vi "water level detection system using arduino.vi"() -> ()   [LabVIEW 2022 SP3]
uses:
  <vilib>/MakerHub/LINX/Public/Peripherals/Analog/Analog Read 1 Chan.vi
  <vilib>/MakerHub/LINX/Public/Peripherals/Digital/Digital Write 1 Chan.vi
  <vilib>/MakerHub/LINX/Public/Peripherals/Analog/Analog Read N Chans.vi
  <vilib>/MakerHub/LINX/Public/Peripherals/Digital/Digital Write N Chans.vi
  <vilib>/MakerHub/LINX/Private/Local IO/LinxAnalogRead.vi
  <vilib>/MakerHub/LINX/Public/Utilities/Check Channel.vi
  <vilib>/MakerHub/LINX/Private/Local IO/LinxDigitalWrite.vi
  <vilib>/MakerHub/LINX/Public/Utilities/Open Serial.vi
  <vilib>/MakerHub/LINX/Private/Utilties/Generate Error.vi
  <vilib>/MakerHub/LINX/LMH-LINX.lvlib
panel:
  out "Boolean 4":bool
  out "Boolean 3":bool
  out "Boolean 2":bool
  out "Boolean":bool
  in  "DO Channel 4":u8
  in  "DO Channel 3":u8
  in  "DO Channel 2":u8
  in  "DO Channel":u8
  in  "stop":bool
  out "Tank":dbl(slide) scale=0.0..10.0
  out "Voltage":dbl
  in  "Analog Channel":u8
  in  "Serial Port":refnum<visa-resource-name>="N/A"
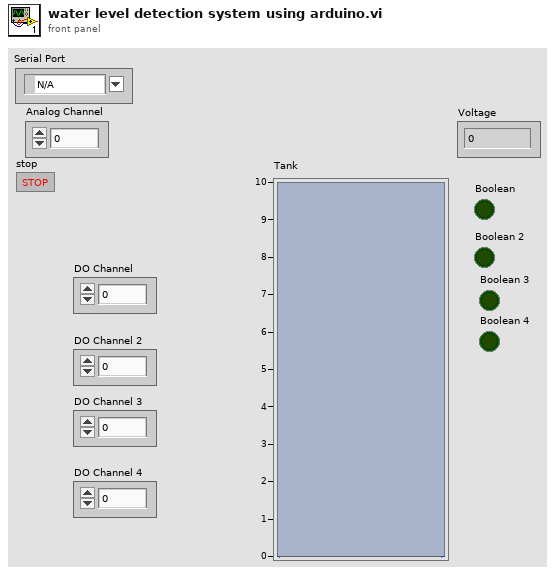
[diagram p1: front panel]
types:
  T1 = typedef "LMH-LINX.lvlib/LINX Ref.ctl" = cluster{"IO":T2, "Interface":T3, "LINX Device Config":T4}
  T2 = typedef "LMH-LINX.lvlib/Platform.ctl" = enum16{"Remote", "Local"}
  T3 = typedef "LMH-LINX.lvlib/Interface.ctl" = enum16{"Serial", "TCP"}
  T4 = typedef "LMH-LINX.lvlib/Device.lvlib/LINX Device Config.ctl" = cluster{"Interface":T3, "COM Port":refnum<visa-resource-name>, "TCP Configuration":T5, "Device Family":u8, "Device ID":u8, "Device Name":string, "TCP Ref":refnum<k5>, "Channels":T6}
  T5 = typedef "LMH-LINX.lvlib/Device.lvlib/TCP Config.ctl" = cluster{"IP Address":string, "Port":u16}
  T6 = typedef "LMH-LINX.lvlib/Channels.ctl" = cluster{"DI":u8[], "DO":u8[], "AI":u8[], "AO":u8[], "PWM":u8[], "QE":u8[], "UART":u8[], "I2C 2":u8[], "SPI":u8[], "CAN":u8[], "Servo":u8[], "AI Ref (V)":dbl, "AI Resolution (Bits)":u8, "AO Ref (V)":dbl, "AO Resolution (Bits)":u8}
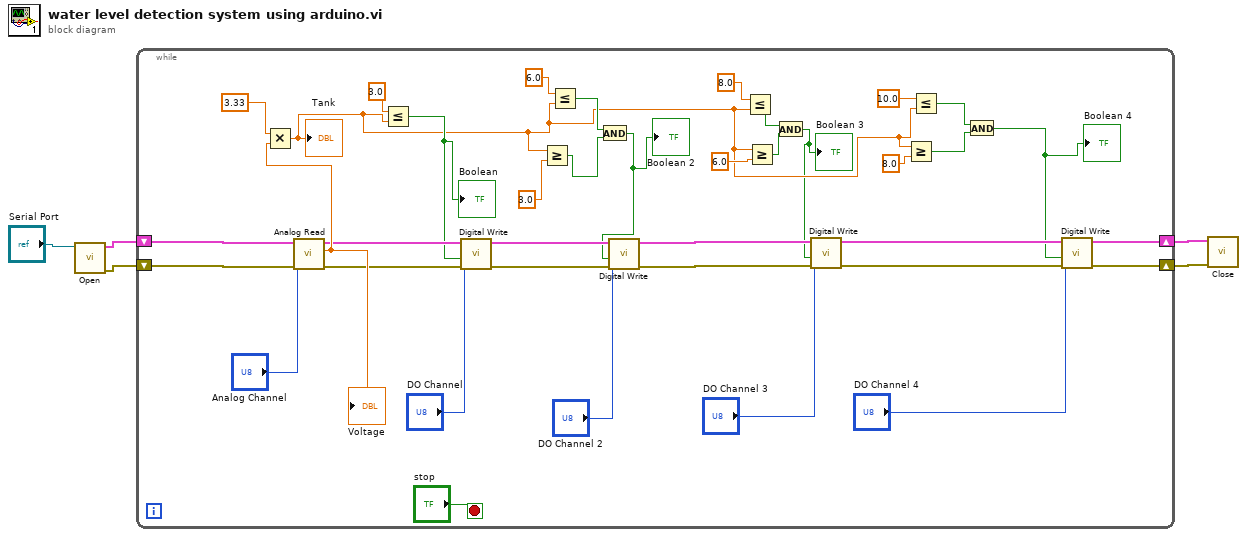
[diagram p0: block diagram]
diagram:
  n1 = call-poly <vilib>:"Open.vi"("Serial Port"="Serial Port") -> ("Error Out"=w3:errorcluster, "LINX Resource"=w4:T1)  [unwired: 8 in, 1 out]
  n2 = while {
    shift-right: [w29] -> w2
    shift-left: w4 -> [w43]
    shift-right: [w28] -> w1
    shift-left: w3 -> [w42]
    stop <- "stop" stop-if-true
    n3 = call-poly <vilib>:"Analog Read.vi"("Error In"=w42, "Analog Channel"="Analog Channel", "LINX Resource"=w43) -> ("Error Out"=w36:errorcluster, "Voltage"=w39:dbl, "LINX Resource"=w37:T1)  [unwired: 5 in, 1 out]
    "Voltage" <- w39
    n4 = Multiply(x=3.33, y=w39) -> (x*y=w10:dbl)
    "Tank" <- w10
    n5 = Less Or Equal?(x=3.0 ("first"), y=w10) -> (x <= y?=w22:bool)
    "Boolean" <- w22
    n6 = call-poly <vilib>:"Digital Write.vi"("Error In"=w36, "Output Value"=w22, "DO Channel"="DO Channel", "LINX Resource"=w37) -> ("Error Out"=w34:errorcluster, "LINX Resource"=w35:T1)  [unwired: 6 in]
    n7 = Greater Or Equal?(x=w10, y=3.0) -> (x >= y?=w18:bool)
    n8 = Less Or Equal?(x=6.0, y=w10) -> (x <= y?=w19:bool)
    n9 = And(x=w19, y=w18) -> (x .and. y?=w17:bool)
    "Boolean 2" <- w17
    n10 = call-poly <vilib>:"Digital Write.vi"("Error In"=w34, "Output Value"=w17, "DO Channel"="DO Channel 2", "LINX Resource"=w35) -> ("Error Out"=w32:errorcluster, "LINX Resource"=w33:T1)  [unwired: 6 in]
    n11 = Less Or Equal?(x=8.0 ("x 2"), y=w10) -> (x <= y?=w14:bool)
    n12 = Greater Or Equal?(x=w10, y=6.0) -> (x >= y?=w13:bool)
    n13 = And(x=w14, y=w13) -> (x .and. y?=w9:bool)
    "Boolean 3" <- w9
    n14 = call-poly <vilib>:"Digital Write.vi"("Error In"=w32, "Output Value"=w9, "DO Channel"="DO Channel 3", "LINX Resource"=w33) -> ("Error Out"=w30:errorcluster, "LINX Resource"=w31:T1)  [unwired: 6 in]
    n15 = Greater Or Equal?(x=w10, y=8.0) -> (x >= y?=w7:bool)
    n16 = Less Or Equal?(x=10.0, y=w10) -> (x <= y?=w8:bool)
    n17 = And(x=w8, y=w7) -> (x .and. y?=w6:bool)
    "Boolean 4" <- w6
    n18 = call-poly <vilib>:"Digital Write.vi"("Error In"=w30, "Output Value"=w6, "DO Channel"="DO Channel 4", "LINX Resource"=w31) -> ("Error Out"=w28:errorcluster, "LINX Resource"=w29:T1)  [unwired: 6 in]
  }
  n19 = call <vilib>:"Close.vi"("Error In"=w1, "LINX Resource"=w2) -> ()  [unwired: 9 in, 1 out]
